vi "Fgv_acessos.vi"(8 "error in":errorcluster, 10 "Tipo":enum16{"Write", "Read"}(ring), 11 "Log in _acesso":bool) -> (0 "Error out":errorcluster, 3 "Acesso permitido":bool)   [LabVIEW 2016]
panel:
  out "Main_leitura":bool
  # "login"
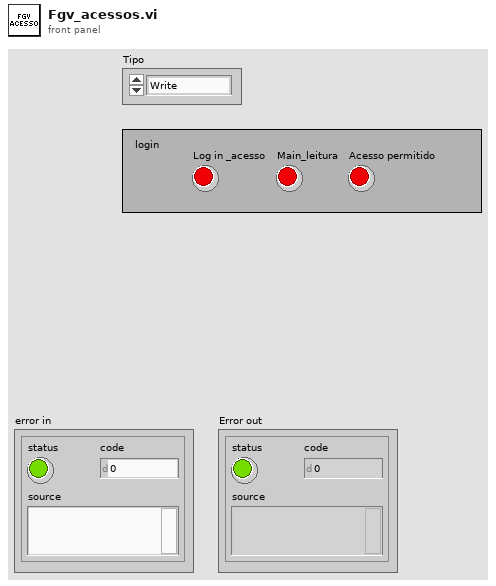
[diagram p1: front panel]
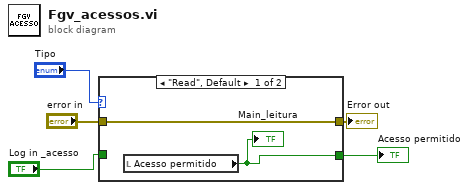
[diagram p0: block diagram]
diagram:
  n1 = case shown="\"Read\", Default" "Tipo" {
    tunnel: "Log in _acesso" -> [_ w8]
    tunnel: [w6 w9] -> w4
    tunnel: "error in" -> [w6 w9]
    tunnel: [w7 w8] -> w1
    frame "Read", Default {
      n2 = local read "Acesso permitido"() -> (w7:bool)
      "Main_leitura" <- w7
    }
    frame "Write" {
    }
  }
  "Error out" <- w4
  "Acesso permitido" <- w1
